vi "Decode Literal Packet.vi"(11 "Bit Stream In":bool[](array[boolean])) -> (2 "Data":u64, 3 "Bit Stream Out":bool[](array[boolean]))   [LabVIEW 2019, in "Day 16.lvlib"]
uses:
  Day 16.lvlib
panel:
  out "Data Groups":bool[][](array[boolean])
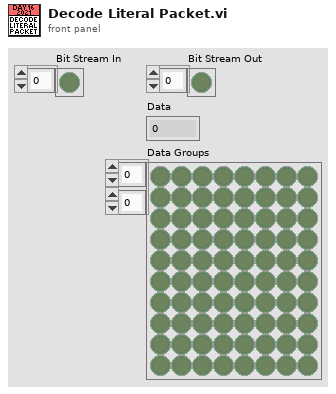
[diagram p1: front panel]
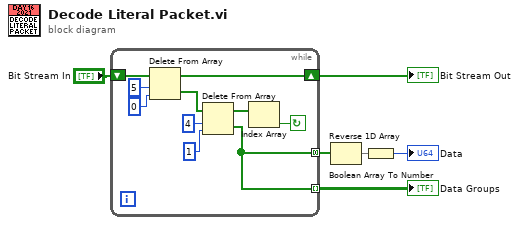
[diagram p0: block diagram]
diagram:
  n1 = while {
    shift-right: [w13] -> w2
    shift-left: "Bit Stream In" -> [w16]
    tunnel: [w9] -> w4 mode=concatenating
    tunnel: [w9] -> w3 mode=indexing
    stop <- w7 continue-if-true
    n2 = Delete From Array(array=w16, length=5, index=0) -> (deleted portion=w14:bool[], array with subset deleted=w13:bool[])
    n3 = Delete From Array(array=w14, length=4, index=1) -> (deleted portion=w9:bool[], array with subset deleted=w10:bool[])
    n4 = Index Array(array=w10) -> (element=w7:bool)  [unwired: 1 in]
  }
  "Data Groups" <- w3
  "Bit Stream Out" <- w2
  n5 = Reverse 1D Array(array=w4) -> (reversed array=w5:bool[])
  n6 = Boolean Array To Number(Boolean array=w5) -> (number=→"Data":u64)
